vi "Upload Score.vi"(8 "error in (no error)":errorcluster, 9 "status":string, 10 "submission":i32, 11 "Run Time":dbl) -> (0 "error out":errorcluster, 2 "Response":string, 5 "Profile URL":string)   [LabVIEW 2024, in "Word Search Scorer.lvlib"]
uses:
  Word Search Scorer.lvlib
  Score Post.ctl
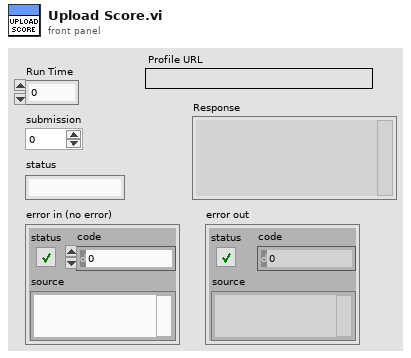
[diagram p1: front panel]
types:
  T1 = typedef "Word Search Scorer.lvlib/Score Post.ctl" = cluster{"scorer":string, "key":string, "submission":i32, "score":dbl, "status":string}
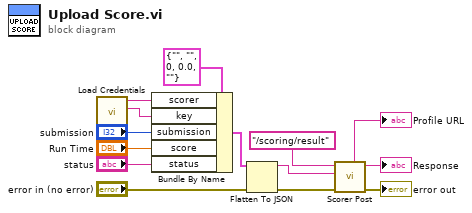
[diagram p0: block diagram]
diagram:
  n1 = call "Load Credentials.vi"() -> ("Key"=w7:string, "ID"=w8:string)  [unwired: 9 in, 1 out]
  n2 = Bundle By Name(cluster=T1 {"scorer"="", "key"="", "submission"=0, "score"=0.0, "status"=""} ("Score Upload"), "scorer"=w8, "key"=w7, "submission"="submission", "score"="Run Time", "status"="status") -> (w6:T1)
  n3 = Flatten To JSON(anything=w6, error in (no error)="error in (no error)") -> (JSON string=w3:string, 11:w4:errorcluster)  [unwired: 1 in]
  n4 = call "Scorer Post.vi"("error in (no error)"=w4, "buffer"=w3, "Path"="/scoring/result") -> ("error out"=→"error out":errorcluster, "Content"=→"Response":string, "Profile URL"=→"Profile URL":string)  [unwired: 5 in, 1 out]
